vi "BiFuncHelp_MatrixMult_CoerceSizeB.vi"(9 "B":T1, 10 "A":T1, 11 "Variant":variant) -> (0 "Error":bool, 3 "Output":T1)   [LabVIEW 2019, in "Trajectory_Library.lvlib"]
uses:
  Trajectory_Library.lvlib
  <vilib>/Analysis/Matrix/Datatypes/RealMatrix.ctl
  <vilib>/Analysis/baseanly.llb/Real A x B.vi
  <vilib>/Analysis/NI_AALBase.lvlib
  <vilib>/Analysis/Matrix/NI_Matrix.lvlib
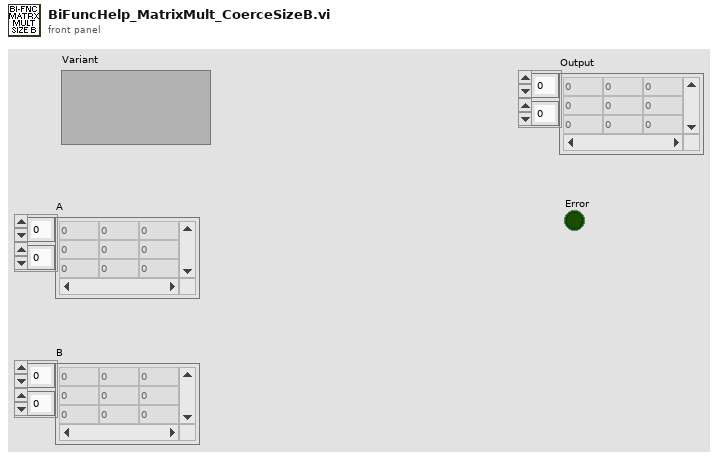
[diagram p1: front panel]
types:
  T1 = typedef "NI_Matrix.lvlib/RealMatrix.ctl" = dbl[][]
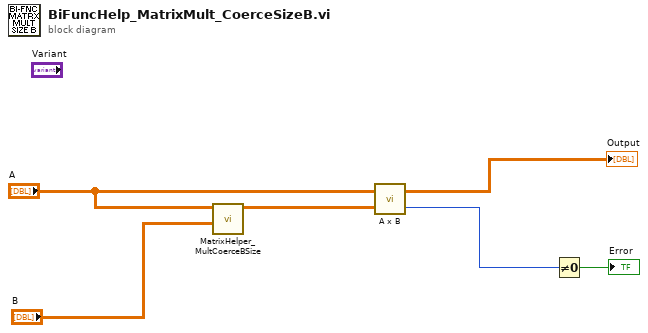
[diagram p0: block diagram]
diagram:
  n1 = call "MatrixHelper_MultCoerceBSize.vi"("B"="B", "A"="A") -> ("Updated B"=w2:T1)  [unwired: 9 in]
  n2 = call-poly <vilib>:"A x B.vi"("B"=w2, "A"="A") -> ("error"=w5:i32, "A x B"=→"Output":T1)
  n3 = Not Equal To 0?(x=w5) -> (x != 0?=→"Error":bool)
